vi "Zeile-Darstellen.vi"(1 "Zeile":i32, 2 "Anfangsspalte":i32, 3 "Anzahl der Elemnte":i32, 4 "Array":string[][](array[string])) -> (0 "String":string)   [LabVIEW 2017]
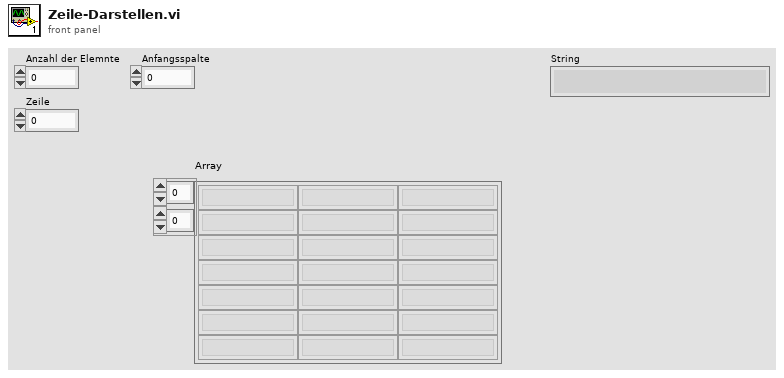
[diagram p1: front panel]
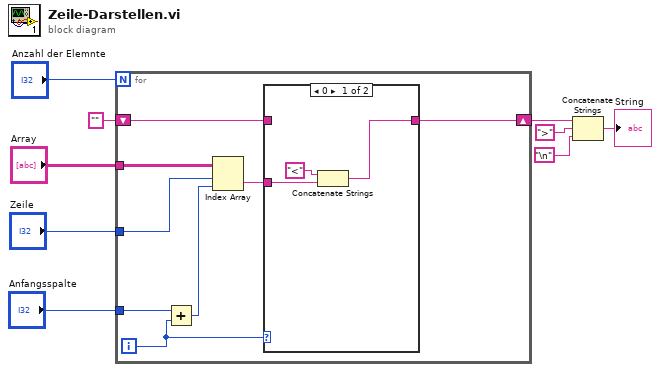
[diagram p0: block diagram]
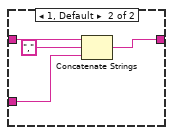
[diagram p2: hidden frame]
diagram:
  n1 = for {
    N: "Anzahl der Elemnte" -> [_]
    tunnel: "Array" -> [w17]
    shift-right: [w16] -> w4
    shift-left: "" -> [w10]
    tunnel: "Zeile" -> [w14]
    tunnel: "Anfangsspalte" -> [w13]
    i -> [w12]
    n2 = Add(x=w13, y=w12) -> (x+y=w11:i32)
    n3 = Index Array(array=w17, index (row)=w14, index (col)=w11) -> (element=w15:string)
    n4 = case shown="0" w12 {
      tunnel: [w18 w23] -> w16
      tunnel: w15 -> [w19 w22]
      tunnel: w10 -> [_ w21]
      frame 0 {
        n5 = Concatenate Strings("<", w19) -> (w18:string)
      }
      frame 1, Default {
        n6 = Concatenate Strings(w21, ",", w22) -> (w23:string)
      }
    }
  }
  n7 = Concatenate Strings(w4, ">", "\n") -> (→"String":string)
